vi "Copy Library.vi"(8 "error in (no error)":errorcluster, 9 "New Name":string, 10 "Destination Directory":path, 11 "Path to Library":path) -> (0 "error out":errorcluster, 3 "New Library Path":path)   [LabVIEW 2020]
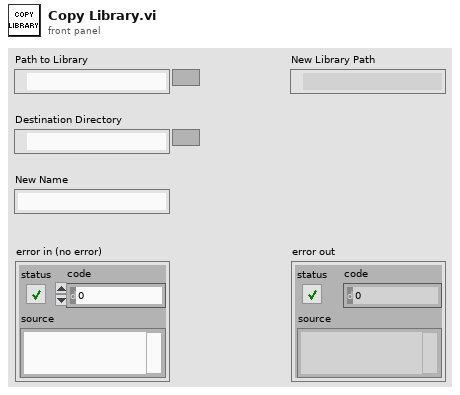
[diagram p1: front panel]
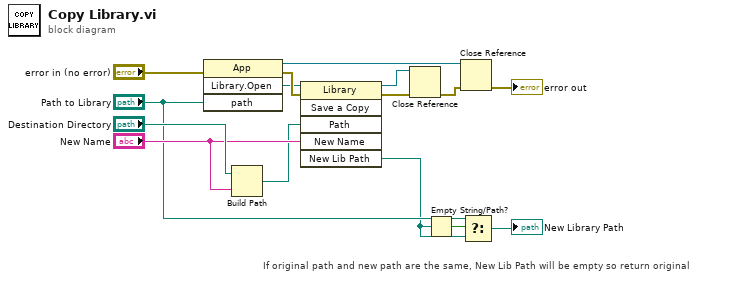
[diagram p0: block diagram]
diagram:
  # "If original path and new path are the same, New Lib Path will be empty so return original"
  n1 = invoke class="App" method="Library.Open"(error in="error in (no error)", "path"="Path to Library") -> (reference out=w10:refnum<vi>, error out=w15:errorcluster, "Open Library"=w14:refnum<vi>)  [unwired: 2 in, 1 out]
  n2 = Build Path(base path="Destination Directory", name or relative path="New Name") -> (appended path=w7:path)
  n3 = invoke class="Library" method="Save a Copy"(reference=w14, error in=w15, "Path"=w7, "New Name"="New Name") -> (reference out=w11:refnum<vi>, error out=w13:errorcluster, "New Lib Path"=w1:path)  [unwired: 2 in, 3 out]
  n4 = Close Reference(reference=w11, error in (no error)=w13) -> (error out=w12:errorcluster)
  n5 = Empty String/Path?(string/path=w1) -> (empty?=w4:bool)
  n6 = Close Reference(reference=w10, error in (no error)=w12) -> (error out=→"error out":errorcluster)
  n7 = Select(t="Path to Library", s=w4, f=w1) -> (s? t:f=→"New Library Path":path)
